vi "Human Interface Pass through.vi"() -> ()   [LabVIEW 2009]
uses:
  <vilib>/userDefined/High Color/nirio_resource_hc.ctl
  <vilib>/rvi/interface/nirviOpenFPGA/nirviOpenFPGA.xnode
  Athena Human Control Code.lvbitx
  <vilib>/FPGAPlugInAG/sbRIO-9642/nirviIntfOpen_sbRIO-9642.vi
  <vilib>/rvi/interface/nirviReadWriteControl/nirviReadWriteControl.xnode
  <vilib>/Utility/error.llb/Error Cluster From Error Code.vi
  <vilib>/rvi/errors/niLvFpgaAdjustHostInterfaceError.vi
  <vilib>/rvi/interface/common/niFpgaNodeNameForErrorReporting.ctl
  <vilib>/rvi/errors/niLvFpgaWhatHappensToTopLevelVI.ctl
  NiRioSrv.dll
  <vilib>/Utility/Variable/NI_VariableUtilities.lvlib
panel:
  out "Right Trigger":i32
  out "Left Trigger":i32
  out "fixed-point":fxp<+/-,32,32>
  out "x*y":fxp<+/-,18,8> format="%.13g"
  out "x/y":fxp<+/-,32,16> format="%.21g"
  out "Left Joy Y-Axis":i32
  out "Left Joy X-Axis":i32
  out "error out":errorcluster
  in  "resource name":T1
  in  "Scale steering by factor of two":i32
  in  "Steering Proportional Control Feedback Gain":fxp<+/-,20,5> format="%.17g"
  out "Throttle Out":fxp<+/-,18,8> format="%.13g"
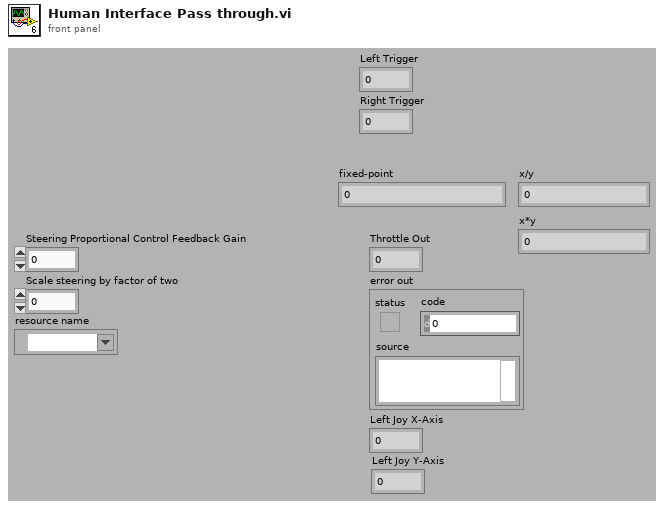
[diagram p1: front panel]
types:
  T1 = typedef "nirio_resource_hc.ctl" = tag
  T2 = typedef "niFpgaNodeNameForErrorReporting.ctl" = enum16{"Open FPGA VI Reference", "Read/Write Control", "Invoke Method: Abort", "Invoke Method: Acknowledge IRQ", "Invoke Method: Download", "Invoke Method: FIFO.Configure", "Invoke Method: FIFO.Read", "Invoke Method: FIFO.Start", "Invoke Method: FIFO.Stop", "Invoke Method: FIFO.Write", "Invoke Method: Reset", "Invoke Method: Run", "Invoke Method: Wait on IRQ", "Close FPGA VI Reference"}
  T3 = typedef "niLvFpgaWhatHappensToTopLevelVI.ctl" = enum16{"top level VI scripted behind XNode", "top level VI inlined behind XNode"}
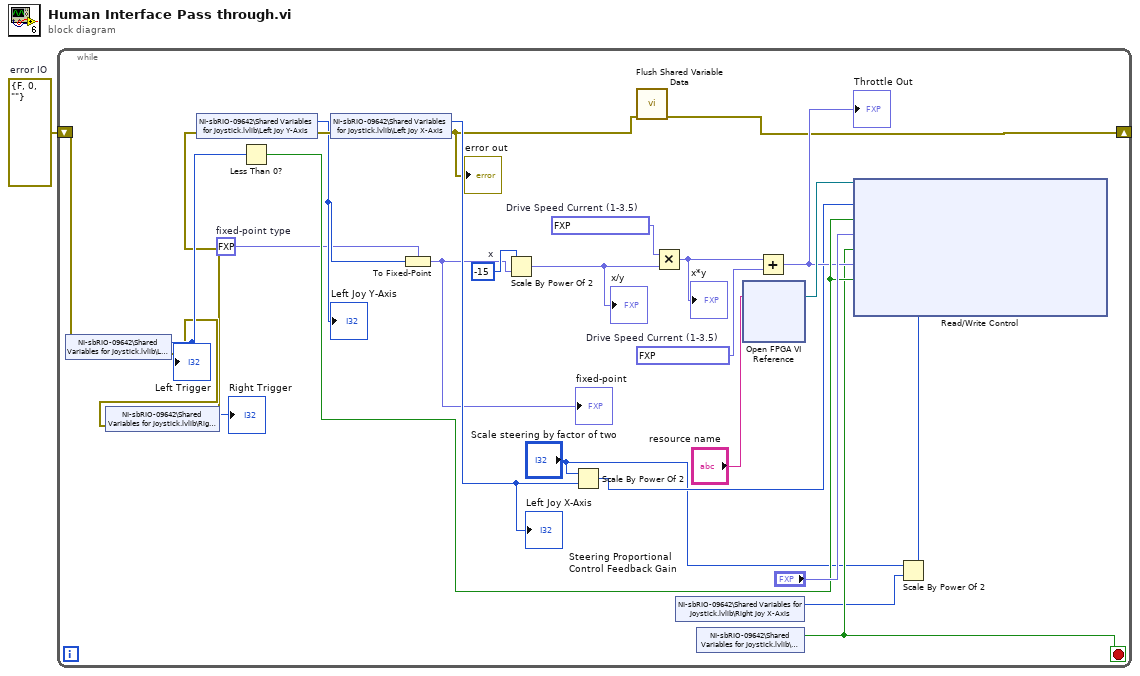
[diagram p0: block diagram]
diagram:
  w1 = errorcluster {"status"=FALSE, "code"=0, "source"=""}  # error IO
  n1 = while {
    shift-right: [w2] -> _
    shift-left: w1 -> [w15]
    stop <- w17 stop-if-true
    w12 = fxp<+/-,32,16> 0.0  # fixed-point type
    w13 = i16 -15  # x
    w22 = fxp<+/-,18,8> -2.5  # Drive Speed Current (1-3.5)
    w25 = fxp<+/-,18,8> 1.0  # Drive Speed Current (1-3.5)
    n2 = shared-variable "NI-sbRIO-09642\\Shared Variables for Joystick.lvlib\\Left Trigger"(error in=w15) -> (w27:i32, error out=w9:errorcluster)
    "Left Trigger" <- w27
    n3 = shared-variable "NI-sbRIO-09642\\Shared Variables for Joystick.lvlib\\Right Trigger"(error in=w9) -> (→"Right Trigger":i32, error out=w8:errorcluster)
    n4 = shared-variable "NI-sbRIO-09642\\Shared Variables for Joystick.lvlib\\Left Joy Y-Axis"(error in=w8) -> (w14:i32, error out=w16:errorcluster)
    "Left Joy Y-Axis" <- w14
    n5 = Less Than 0?(x=w27) -> (x < 0?=w24:bool)
    n6 = shared-variable "NI-sbRIO-09642\\Shared Variables for Joystick.lvlib\\Left Joy X-Axis"(error in=w16) -> (w20:i32, error out=w3:errorcluster)
    "error out" <- w3
    "Left Joy X-Axis" <- w20
    n7 = To Fixed-Point(fixed-point type=w12, number=w14) -> (fixed-point=w10:fxp<+/-,32,16>)
    "fixed-point" <- w10
    n8 = Scale By Power Of 2(n=w13, x=w10) -> (x*2^n=w11:fxp<+/-,32,16>)
    "x/y" <- w11
    n9 = Scale By Power Of 2(n="Scale steering by factor of two", x=w20) -> (x*2^n=w19:i32)
    n10 = call <vilib>:"Flush Shared Variable Data.vi"("error in (no error)"=w3) -> ("error out"=w2:errorcluster)  [unwired: 10 in]
    n11 = Multiply(x=w22, y=w11) -> (x*y=w21:fxp<+/-,18,8>)
    "x*y" <- w21
    n12 = shared-variable "NI-sbRIO-09642\\Shared Variables for Joystick.lvlib\\Right Joy X-Axis"() -> (w5:i32)  [unwired: 1 in, 1 out]
    n13 = shared-variable "NI-sbRIO-09642\\Shared Variables for Joystick.lvlib\\Start Button"() -> (w17:bool)  [unwired: 1 in, 1 out]
    n14 = xnode "Open FPGA VI Reference"("resource name"="resource name") -> ("FPGA VI Reference Out"=w28:refnum<k20>)  [unwired: 1 in, 1 out]
    n15 = Add(x=w21, y=w25) -> (x+y=w23:fxp<+/-,18,8>)
    "Throttle Out" <- w23
    n16 = Scale By Power Of 2(n="Scale steering by factor of two", x=w5) -> (x*2^n=w6:i32)
    n17 = xnode "Read/Write Control"("FPGA VI Reference In"=w28, "Steering Position Target"=w19, "Steering Enable"=w24, "Steering Proportional Control Feedback Gain"="Steering Proportional Control Feedback Gain", "Stop"=w17, "Drive Speed Current (1-3.5)"=w23, "Drive Enable"=w24, "Steering Position Offset"=w6) -> ()  [unwired: 1 in, 3 out]
  }
